vi "Kalman_gain.vi"(9 "R":T1, 10 "Jk":T1, 11 "Pk":T1) -> (3 "K":T1)   [LabVIEW 2019]
uses:
  <vilib>/Analysis/Matrix/Datatypes/RealMatrix.ctl
  <vilib>/Analysis/baseanly.llb/Real A x B.vi
  <vilib>/Analysis/Matrix/Numeric/Add/Add - RM,RM.vi
  <vilib>/Analysis/baseanly.llb/Real Inverse Matrix.vi
  <vilib>/Analysis/NI_AALBase.lvlib
  <vilib>/Analysis/Matrix/NI_Matrix.lvlib
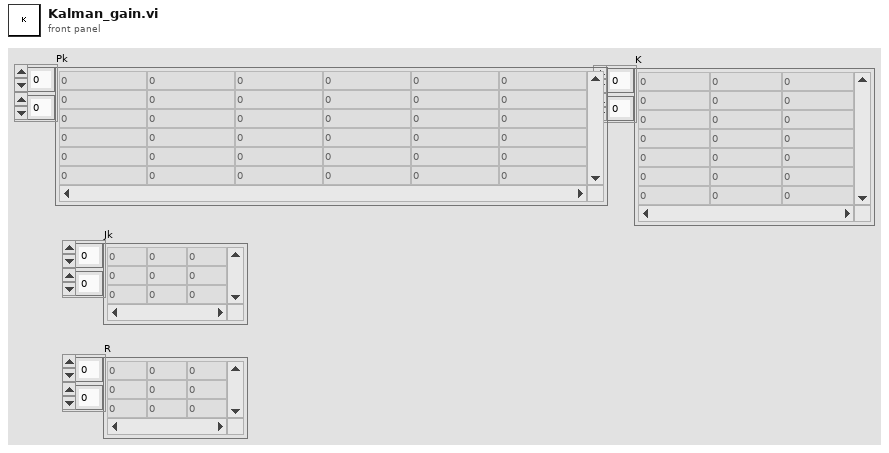
[diagram p1: front panel]
types:
  T1 = typedef "NI_Matrix.lvlib/RealMatrix.ctl" = dbl[][]
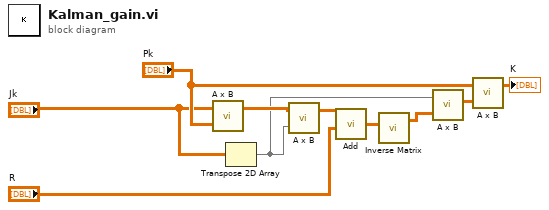
[diagram p0: block diagram]
diagram:
  n1 = call-poly <vilib>:"A x B.vi"("B"="Pk", "A"="Jk") -> ("A x B"=w2:T1)  [unwired: 1 out]
  n2 = Transpose 2D Array(2D array="Jk") -> (transposed array=w1:T1)
  n3 = call-poly <vilib>:"A x B.vi"("B"=w1, "A"=w2) -> ("A x B"=w4:T1)  [unwired: 1 out]
  n4 = call-poly <vilib>:"Add.vi"("Real Matrix B"="R", "Real Matrix A"=w4) -> ("A + B"=w6:T1)
  n5 = call-poly <vilib>:"Inverse Matrix.vi"("Input Matrix"=w6) -> ("Inverse Matrix"=w7:T1)  [unwired: 1 in, 1 out]
  n6 = call-poly <vilib>:"A x B.vi"("B"=w7, "A"=w1) -> ("A x B"=w8:T1)  [unwired: 1 out]
  n7 = call-poly <vilib>:"A x B.vi"("B"=w8, "A"="Pk") -> ("A x B"=→"K":T1)  [unwired: 1 out]
